vi "z closure query call.vi"(8 "error in (no error)":errorcluster, 10 "query":cluster{}, 11 "closure":cluster{}) -> (0 "error out":errorcluster, 2 "query out":cluster{})   [LabVIEW 2021, in "zenohc.lvlib"]
doc: "void z_closure_query_call(const struct z_loaned_closure_query_t *closure,\n struct z_loaned_query_t *query);"
uses:
  zenohc.lvlib
  zenohc.dll
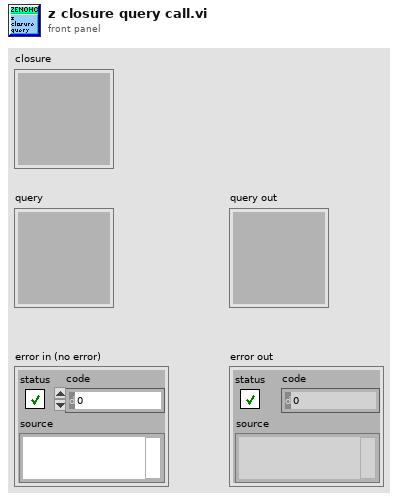
[diagram p1: front panel]
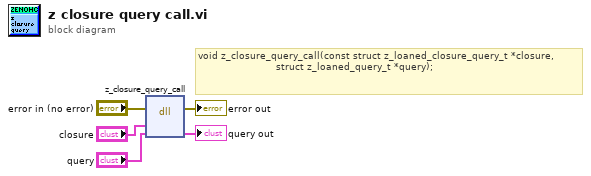
[diagram p0: block diagram]
diagram:
  # "void z_closure_query_call(const struct z_loaned_closure_query_t *closure,\n                          struct z_loaned_query_t *query);"
  n1 = dll-call lib="D:/dev/zenoh_labview/zenohc/zenohc.*" fn="z_closure_query_call"(error in="error in (no error)", "closure"="closure", "query"="query") -> (error out=→"error out":errorcluster, "query"=→"query out":cluster{})  [unwired: 4 in, 1 out]
